vi "Get Aperture Time.vi"(0 "Instrument handle IN":refnum<k15>[](array[refnum]), 5 "Channel Name":string[](array[string]), 7 "Minimum Sequence dt(s)":dbl[](array[numeric]), 9 "Measure Period":dbl=0.001 format="%#.3p", 11 "error in (no error)":errorcluster) -> (4 "Instrument handle OUT":refnum<k15>[](array[refnum]), 6 "Aperture Time":dbl[](array[numeric]), 15 "error out":errorcluster)   [LabVIEW 2024, in "devicePowerSequencerCoreLogic.lvlib"]
uses:
  devicePowerSequencerCoreLogic.lvlib
  <vilib>/Utility/config.llb/Read Key (Double).vi
  <vilib>/Utility/config.llb/NI_LVConfig.lvlib
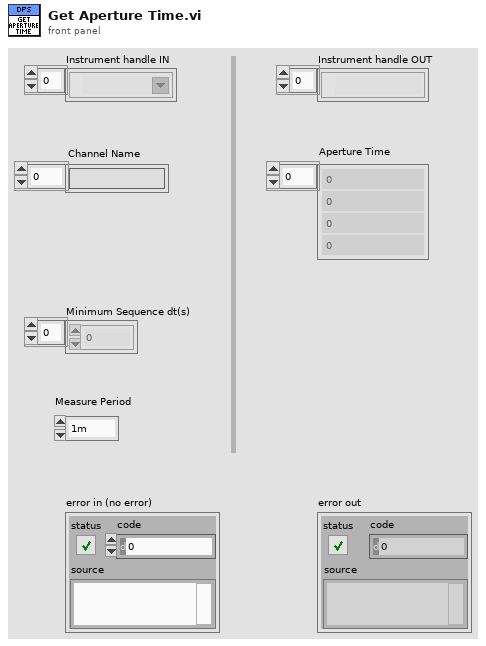
[diagram p1: front panel]
types:
  T1 = typedef "NI_LVConfig.lvlib/Config Data RefNum.ctl" = refnum<k1>
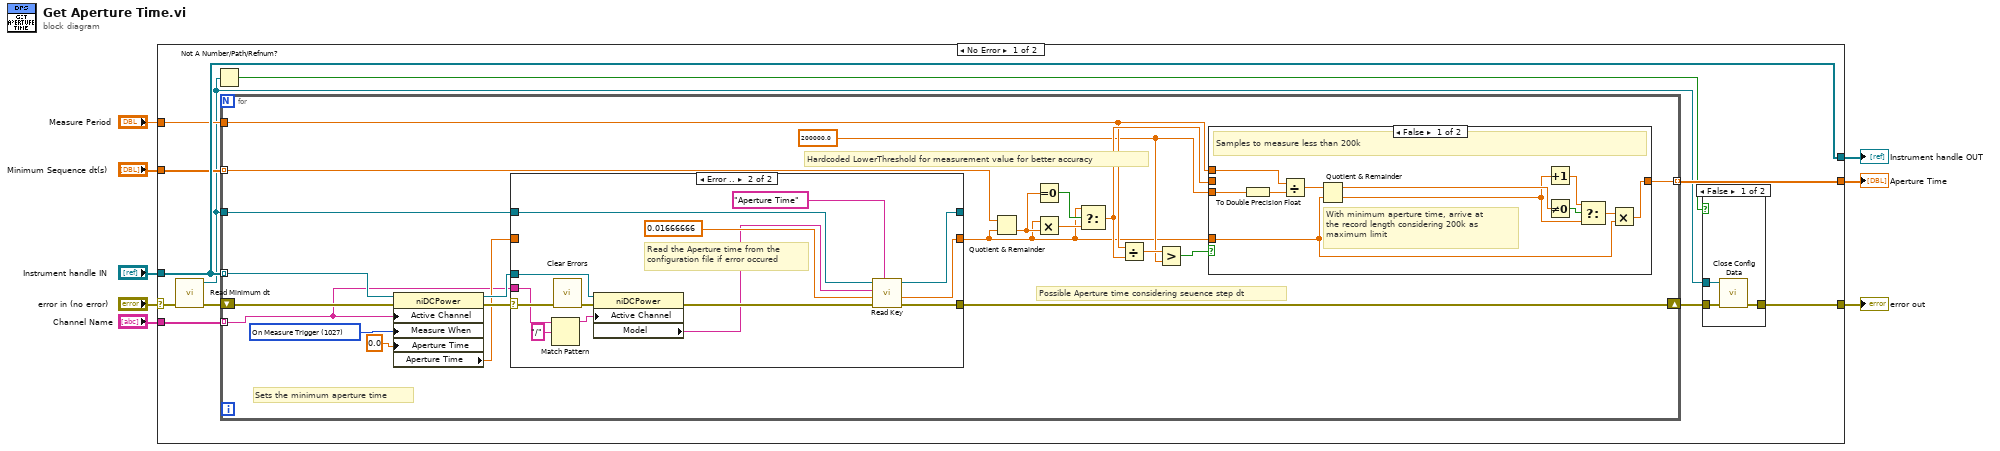
[diagram p0: block diagram]
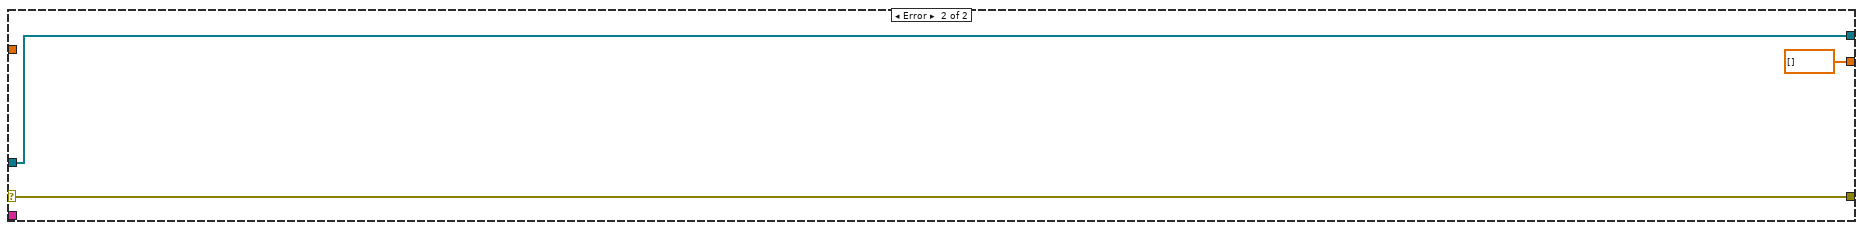
[diagram p5: hidden frame]
diagram:
  n1 = case shown="No Error" "error in (no error)" {
    selector: "error in (no error)" -> [w15 w76]
    tunnel: "Instrument handle IN" -> [w19 w74]
    tunnel: [w11 w76] -> w6
    tunnel: [w17 dbl[] []] -> w5
    tunnel: [w19 w74] -> w4
    tunnel: "Channel Name" -> [w18 _]
    tunnel: "Minimum Sequence dt(s)" -> [w16 _]
    tunnel: "Measure Period" -> [w13 _]
    frame No Error {
      n2 = call "Read Minimum dt.vi"("error in (no error)"=w15) -> ("refnum"=w9:T1, "error out"=w14:errorcluster)  [unwired: 12 in, 1 out]
      n3 = Not A Number/Path/Refnum?(number/path/refnum=w9) -> (NaN/Path/Refnum?=w10:bool)
      n4 = for {
        tunnel: w19 -> [w44] mode=indexing
        tunnel: w18 -> [w24] mode=indexing
        shift-right: [w25] -> w12
        shift-left: w14 -> [w43]
        tunnel: [w26] -> w17 mode=indexing
        tunnel: w16 -> [w40] mode=indexing
        tunnel: w9 -> [w36]
        tunnel: w13 -> [w29]
        w28 = 200000.0 ("y")
        w41 = 1027 items=["Automatically after Source Complete"=1025, "On Demand"=1026, "On Measure Trigger"=1027] ("Measurement:Advanced:Measure When")
        # "Hardcoded LowerThreshold for measurement value for better accuracy"
        # "Possible Aperture time considering seuence step dt"
        # "Sets the minimum aperture time"
        n5 = property class="niDCPower"(reference=w44, error in=w43, "Active Channel"=w24, "Measure When"=w41, "Aperture Time"=0.0 ("Measurement:Aperture Time")) -> (reference out=w38:refnum<k15>, error out=w39:errorcluster, "Aperture Time"=w37:dbl)
        n6 = case shown="Error .." w39 {
          selector: w39 -> [w57 w68]
          tunnel: w36 -> [w58 w73]
          tunnel: w38 -> [_ w70]
          tunnel: w37 -> [w59 _]
          tunnel: [w59 w69] -> w27
          tunnel: [w57 w65] -> w25
          tunnel: [w58 w66] -> _
          tunnel: w24 -> [_ w62]
          frame No Error {
            # "Get the minimum aperture time"
          }
          frame Error {
            # "Read the Aperture time from the\nconfiguration file if error occured"
            n7 = Match Pattern(string=w62, regular expression="/") -> (before substring=w60:string)  [unwired: 1 in, 3 out]
            n8 = call <vilib>:"Clear Errors.vi"("error in (no error)"=w68) -> ("error out"=w67:errorcluster)  [unwired: 5 in, 1 out]
            n9 = property class="niDCPower"(reference=w70, error in=w67, "Active Channel"=w60) -> (error out=w71:errorcluster, "Model"=w63:string)  [unwired: 1 out]
            n10 = call-poly <vilib>:"Read Key.vi"("section"="Aperture Time", "error in (no error)"=w71, "default value"=0.01666666, "key"=w63, "refnum"=w73) -> ("error out"=w65:errorcluster, "value"=w69:dbl, "refnum out"=w66:T1)  [unwired: 3 in, 1 out]
          }
        }
        n11 = Quotient & Remainder(x=w40, y=w27) -> (floor(x/y)=w35:dbl)  [unwired: 1 out]
        n12 = Equal To 0?(x=w35) -> (x = 0?=w34:bool)
        n13 = Multiply(x=w27, y=w35) -> (x*y=w33:dbl)
        n14 = Select(t=w27, s=w34, f=w33) -> (s? t:f=w30:dbl)
        n15 = Divide(x=w29, y=w30) -> (x/y=w32:dbl)
        n16 = Greater?(x=w32, y=w28) -> (0:w31:bool)
        n17 = case shown="False" w31 {
          tunnel: w30 -> [_ w56]
          tunnel: [w45 w56] -> w26
          tunnel: w29 -> [w49 _]
          tunnel: w28 -> [w48 _]
          tunnel: w27 -> [w47 _]
          frame False {
            # "With minimum aperture time, arrive at  the record length considering 200k as maximum limit"
            # "Samples to measure less than 200k"
            n18 = To Double Precision Float(number=w48) -> (double precision float=w50:dbl)
            n19 = Divide(x=w49, y=w50) -> (x/y=w55:dbl)
            n20 = Quotient & Remainder(x=w55, y=w47) -> (x-y*floor(x/y)=w54:dbl, floor(x/y)=w52:dbl)
            n21 = Increment(x=w52) -> (x+1=w51:dbl)
            n22 = Not Equal To 0?(x=w54) -> (x != 0?=w53:bool)
            n23 = Select(t=w51, s=w53, f=w52) -> (s? t:f=w46:dbl)
            n24 = Multiply(x=w46, y=w47) -> (x*y=w45:dbl)
          }
          frame True {
            # "Samples to measure greater than 200k"
          }
        }
      }
      n25 = case shown="False" w10 {
        tunnel: w12 -> [w22 w23]
        tunnel: [w21 w23] -> w11
        tunnel: w9 -> [w20 _]
        frame False {
          n26 = call <vilib>:"Close Config Data.vi"("error in (no error)"=w22, "refnum"=w20) -> ("error out"=w21:errorcluster)  [unwired: 8 in, 1 out]
        }
        frame True {
        }
      }
    }
    frame Error {
    }
  }
  "error out" <- w6
  "Instrument handle OUT" <- w4
  "Aperture Time" <- w5
